vi "SineToSquare.vi"() -> ()   [LabVIEW 2019]
panel:
  out "Square wave":dbl[](graph)=[0.0, 2.0, 2.0, 2.0, 2.0, 2.0, 2.0, 2.0, 2.0, 2.0, 2.0, -2.0, -2.0, -2.0, -2.0, -2.0, -2.0, -2.0, -2.0, -2.0, -2.0, 2.0, 2.0, 2.0, 2.0, 2.0, 2.0, 2.0, 2.0, 2.0, 2.0, -2.0, -2.0, -2.0, -2.0, -2.0, -2.0, -2.0, -2.0, -2.0]
  in  "Amplitude":dbl=2.0
  out "Integrated Triangle wave":dbl[](graph)=[0.0, 0.0002, 0.0004, 0.0006000000000000001, 0.0008, 0.001, 0.0012000000000000001, 0.0014000000000000002, 0.0016000000000000003, 0.0018000000000000004, 0.0020000000000000005, 0.0018000000000000004, 0.0016000000000000003, 0.0014000000000000002, 0.0012000000000000001, 0.001, 0.0008, 0.0006000000000000001, 0.0004000000000000001, 0.00020000000000000006, 5.421010862427522e-20, 0.00020000000000000006, 0.0004000000000000001, 0.0006000000000000001, 0.0008, 0.001, 0.0012000000000000001, 0.0014000000000000002, 0.0016000000000000003, 0.0018000000000000004, 0.0020000000000000005, 0.0018000000000000004, 0.0016000000000000003, 0.0014000000000000002, 0.0012000000000000001, 0.001, 0.0008, 0.0006000000000000001, 0.0004000000000000001, 0.00020000000000000006]
  out "Integration\nsum":dbl=0.00020000000000000006
  out "No. of\nsamples":dbl=40.0
  in  "No. of\ncycles":dbl=2.0
  in  "fs":dbl=10000.0
  in  "Phase":dbl
  in  "f":dbl=500.0
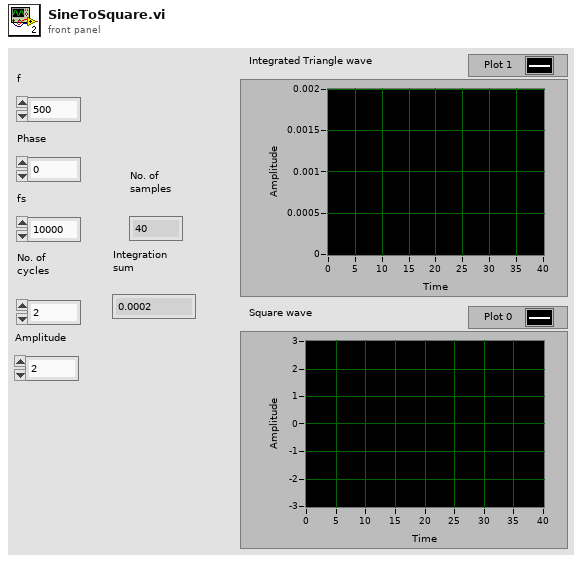
[diagram p1: front panel]
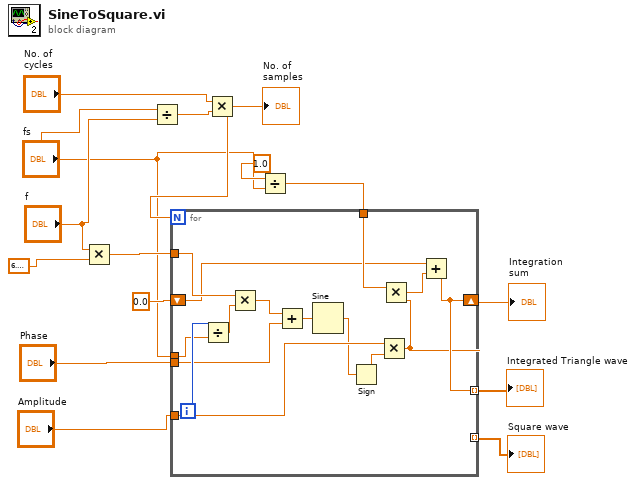
[diagram p0: block diagram]
diagram:
  n1 = Multiply(x="f", y=6.283185307179586) -> (x*y=w8:dbl)
  n2 = Divide(x="fs", y="f") -> (x/y=w15:dbl)
  n3 = Multiply(x="No. of\ncycles", y=w15) -> (x*y=w13:dbl)
  "No. of\nsamples" <- w13
  n4 = Divide(x=1.0, y="fs") -> (x/y=w6:dbl)
  n5 = for {
    N: w13 -> [_]
    tunnel: "fs" -> [w29]
    shift-right: [w19] -> w4
    shift-left: 0.0 ("x") -> [w20]
    tunnel: w8 -> [w27]
    tunnel: "Phase" -> [w25]
    tunnel: w6 -> [w24]
    tunnel: "Amplitude" -> [w23]
    tunnel: [w19] -> w2 mode=indexing
    tunnel: [w16] -> w1 mode=indexing
    i -> [w30]
    n6 = Divide(x=w30, y=w29) -> (x/y=w28:dbl)
    n7 = Multiply(x=w27, y=w28) -> (x*y=w26:dbl)
    n8 = Add(x=w26, y=w25) -> (x+y=w22:dbl)
    n9 = Sine(x=w22) -> (sin(x)=w18:dbl)
    n10 = Sign(1:w18) -> (0:w17:dbl)
    n11 = Multiply(x=w23, y=w17) -> (x*y=w16:dbl)
    n12 = Multiply(x=w24, y=w16) -> (x*y=w21:dbl)
    n13 = Add(x=w20, y=w21) -> (x+y=w19:dbl)
  }
  "Integration\nsum" <- w4
  "Integrated Triangle wave" <- w2
  "Square wave" <- w1
